vi "Disconnect.vi"(8 "error in (no error)":errorcluster, 11 "DelayLineLS4 en entrée":refnum<class "DLLS4.lvclass">) -> (0 "error out":errorcluster, 3 "DelayLineLS4 out":refnum<class "DLLS4.lvclass">)   [LabVIEW 2018, in "DLLS4.lvclass"]
uses:
  DLLS4.lvclass
  C:/Dev/TRANCON/Classes/Delay Line/DelayLine.lvclass
  DelayLine.lvclass/DelayLine.ctl
  <vilib>/Utility/error.llb/DialogType.ctl
  <vilib>/ErrorRing/Error Ring.xnode
  DelayLine.lvclass
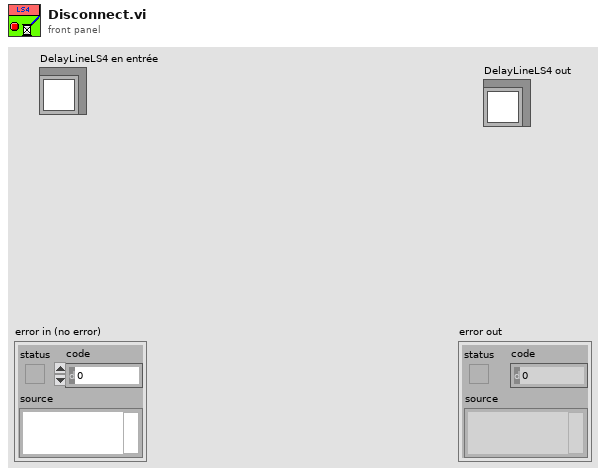
[diagram p1: front panel]
types:
  T1 = typedef "DialogType.ctl" = u16
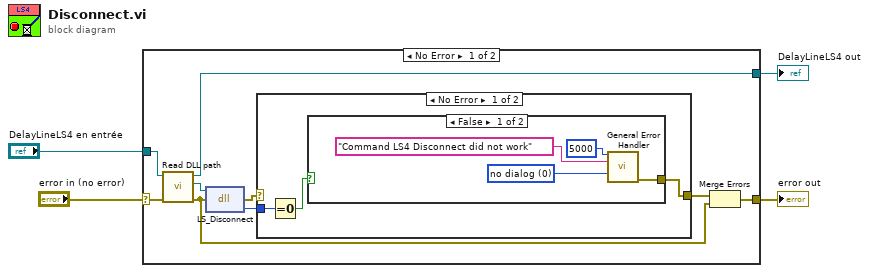
[diagram p0: block diagram]
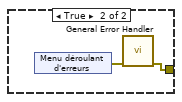
[diagram p2: hidden frame]
diagram:
  n1 = case shown="No Error" "error in (no error)" {
    selector: "error in (no error)" -> [w5 w26]
    tunnel: [w8 w26] -> w3
    tunnel: [w10 w25] -> w1
    tunnel: "DelayLineLS4 en entrée" -> [w6 w25]
    frame No Error {
      n2 = call "Read DLL path.vi"("error in (no error)"=w5, "DelayLine in"=w6) -> ("error out"=w7:errorcluster, "DLL path"=w11:path, "DelayLine out"=w10:refnum<class "DLLS4.lvclass">)  [unwired: 7 in]
      n3 = dll-call lib="S:/TRANCON/DLL/LStep4.dll" fn="LS_Disconnect"(path in=w11, error in=w7) -> (error out=w12:errorcluster, "type de retour"=w13:i32)  [unwired: 1 in, 1 out]
      n4 = case shown="No Error" w12 {
        selector: w12 -> [_ w24]
        tunnel: w13 -> [w16 _]
        tunnel: [w14 w24] -> w9
        frame No Error {
          n5 = Equal To 0?(x=w16) -> (x = 0?=w15:bool)
          n6 = case shown="False" w15 {
            tunnel: [w18 w21] -> w14
            frame False {
              w17 = T1 0 items=["no dialog", "OK message", "continue or stop message", "OK message + warnings", "continue/stop + warnings"] ("type of dialog (OK msg:1)")
              n7 = call <vilib>:"General Error Handler.vi"("[error code] (0)"=5000 ("code"), "[error source] (\" \")"="Command LS4 Disconnect did not work" ("String to Prepend to source (\"\")"), "type of dialog (OK msg:1)"=w17) -> ("error out"=w18:errorcluster)  [unwired: 8 in, 4 out]
            }
            frame True {
              n8 = xnode "Menu déroulant d'erreurs"() -> ("error out"=w22:errorcluster)
              n9 = call <vilib>:"General Error Handler.vi"("error in (no error)"=w22) -> ("error out"=w21:errorcluster)  [unwired: 10 in, 4 out]
            }
          }
        }
        frame Error {
        }
      }
      n10 = Merge Errors(w9, w7) -> (w8:errorcluster)
    }
    frame Error {
    }
  }
  "error out" <- w3
  "DelayLineLS4 out" <- w1
